vi "Control_Rack_Controler.vi"(0 "Times":dbl[](array[numeric]), 1 "Voltages Toroidal (Keep below |10|)":dbl[](array[numeric]), 2 "Voltages Helical (Keep below |10|)":dbl[](array[numeric]), 3 "error out":errorcluster, 4 "Data out 2":T1) -> (5 "error out 2":errorcluster, 6 "Data out":T1)   [LabVIEW 2017]
uses:
  Type_Defs/Data.ctl
  Type_Defs/Diagnostics.ctl
  Type_Defs/Systems.ctl
  <vilib>/DAQmx/write.llb/DAQmx Write (Analog DBL 1Chan 1Samp).vi
  <vilib>/DAQmx/create/channels.llb/DAQmx Create Channel (AO-Voltage-Basic).vi
  <vilib>/DAQmx/miscellaneous.llb/DAQmx Fill In Error Info.vi
  <vilib>/express/express shared/transition.llb/Dynamic To Waveform Array.vi
  <vilib>/express/express signal manip/GetorSetDDTAttributes/Set DDT Attributes/SetT0.vi
  <vilib>/express/express shared/transition.llb/Waveform Array To Dynamic.vi
  <vilib>/express/express signal manip/GetorSetDDTAttributes/Set DDT Attributes/Set DDT Properties.xnode
panel:
  out "hel_cur":dynamicdata(graph) caption="Helix Current Feedback"
  out "hel_vol":dynamicdata(graph) caption="Helix Voltage Feedback"
  out "hel_cur_set":dynamicdata(graph) caption="Helix Limited Current Set Point"
  out "torr_cur_set":dynamicdata(graph) caption="Torroidal Limited Current Set Point"
  out "torr_vol":dynamicdata(graph) caption="Torroidal Voltage Feedback"
  out "torr_cur":dynamicdata(graph) caption="Torroidal Current Feedback"
  out "Voltage Toroidal":dbl
  out "Time":dbl
  out "Voltage Helical":dbl
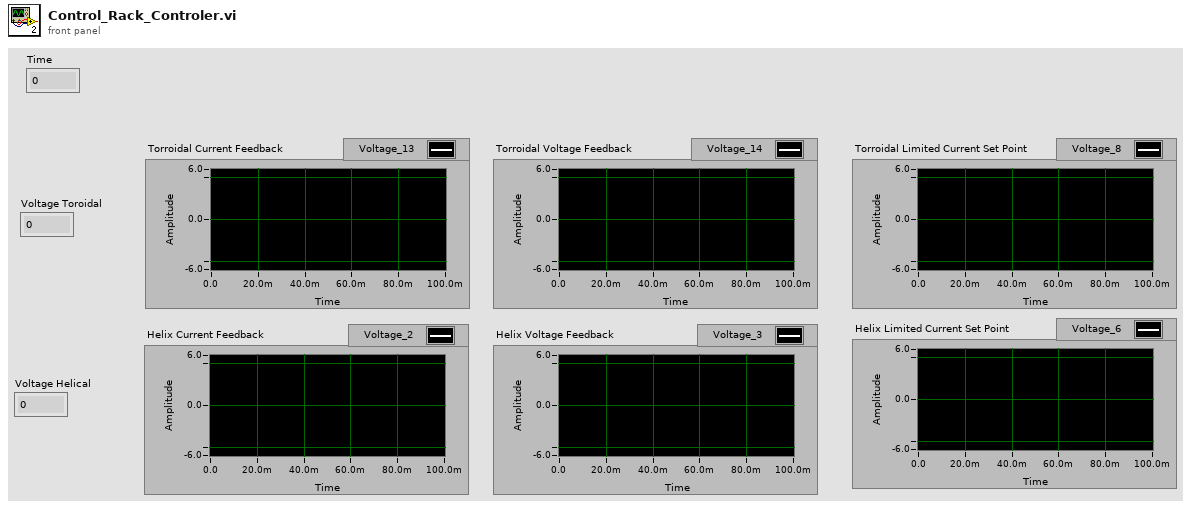
[diagram p1: front panel]
types:
  T1 = typedef "Data.ctl" = cluster{"User Name":string, "Experiment Number":i32, "Start Time":timestamp, "Data":dbl[], "Step Number":i32, "Step Instructions":string, "Diagnostics":T2, "Experiment Purpose":string, "Experiment State":enum16{"Off", "Setting Up", "Ready", "In Progress", "Shutting Down"}, "Systems":T3, "Vacuum Pressure":dbl, "Fieldpoints":cluster{"System Boolean Fieldpoints":cluster{"Compressed Air":refnum<k21>, "T-20kV Power Switch":refnum<k21>, "T-Rectifier":refnum<k21>, "Engage Interlock":refnum<k21>, "Ventilator":refnum<k21>, "Magnetron":refnum<k21>, "H-20kV Power Switch":refnum<k21>, "H-Rectifier":refnum<k21>, "Main Water Pump":refnum<k21>, "WEGA Water Pump":refnum<k21>, "Gas Inlet Valves":refnum<k21>}, "Step Fieldpoints":cluster{"Exhaust Ventillator":refnum<k21>, "Compressed Air":refnum<k21>, "Water Pressure":refnum<k21>, "Interlock":refnum<k21>, "Toroidal Power Supply 1":refnum<k21>, "Toroidal Power Supply 2":refnum<k21>, "Toroidal Rectifier":refnum<k21>, "Helical Power Supply":refnum<k21>, "Helical Rectifier":refnum<k21>, "6kW Magnetron Standby":refnum<k21>, "20kW Magnetron Standby":refnum<k21>}}, "Pressure History":cluster{"Seconds into Experiment":i32[], "Pressure Data":dbl[]}, "Time Computer Control":dbl[], "Toroidal Voltage Computer Control":dbl[], "Helical Voltage Computer Control":dbl[], "Toroidal Current":dbl[], "Toroidal Voltage":dbl[], "Toroidal Current Set Point":dbl[], "Helical Current Set Point":dbl[], "Helical Voltage":dbl[], "Helical Current":dbl[], "Experiment Folder":path, "Run Another Shot?":bool}
  T2 = typedef "Diagnostics.ctl" = cluster{"Langmuir Probe":bool, "Rogowski 1":bool, "Rogowski 2":bool, "Rogowski 3":bool, "B-dot 1":bool, "B-dot 2":bool}
  T3 = typedef "Systems.ctl" = cluster{"Compressed Air":bool, "T-20kV Power Switch":bool, "T-Rectifier":bool, "Engage Interlock":bool, "Ventilator":bool, "Magnetron":bool, "H-20kV Power Switch":bool, "H-Rectifier":bool, "Main Water Pump":bool, "WEGA Water Pump":bool, "Gas Inlet Valves":bool}
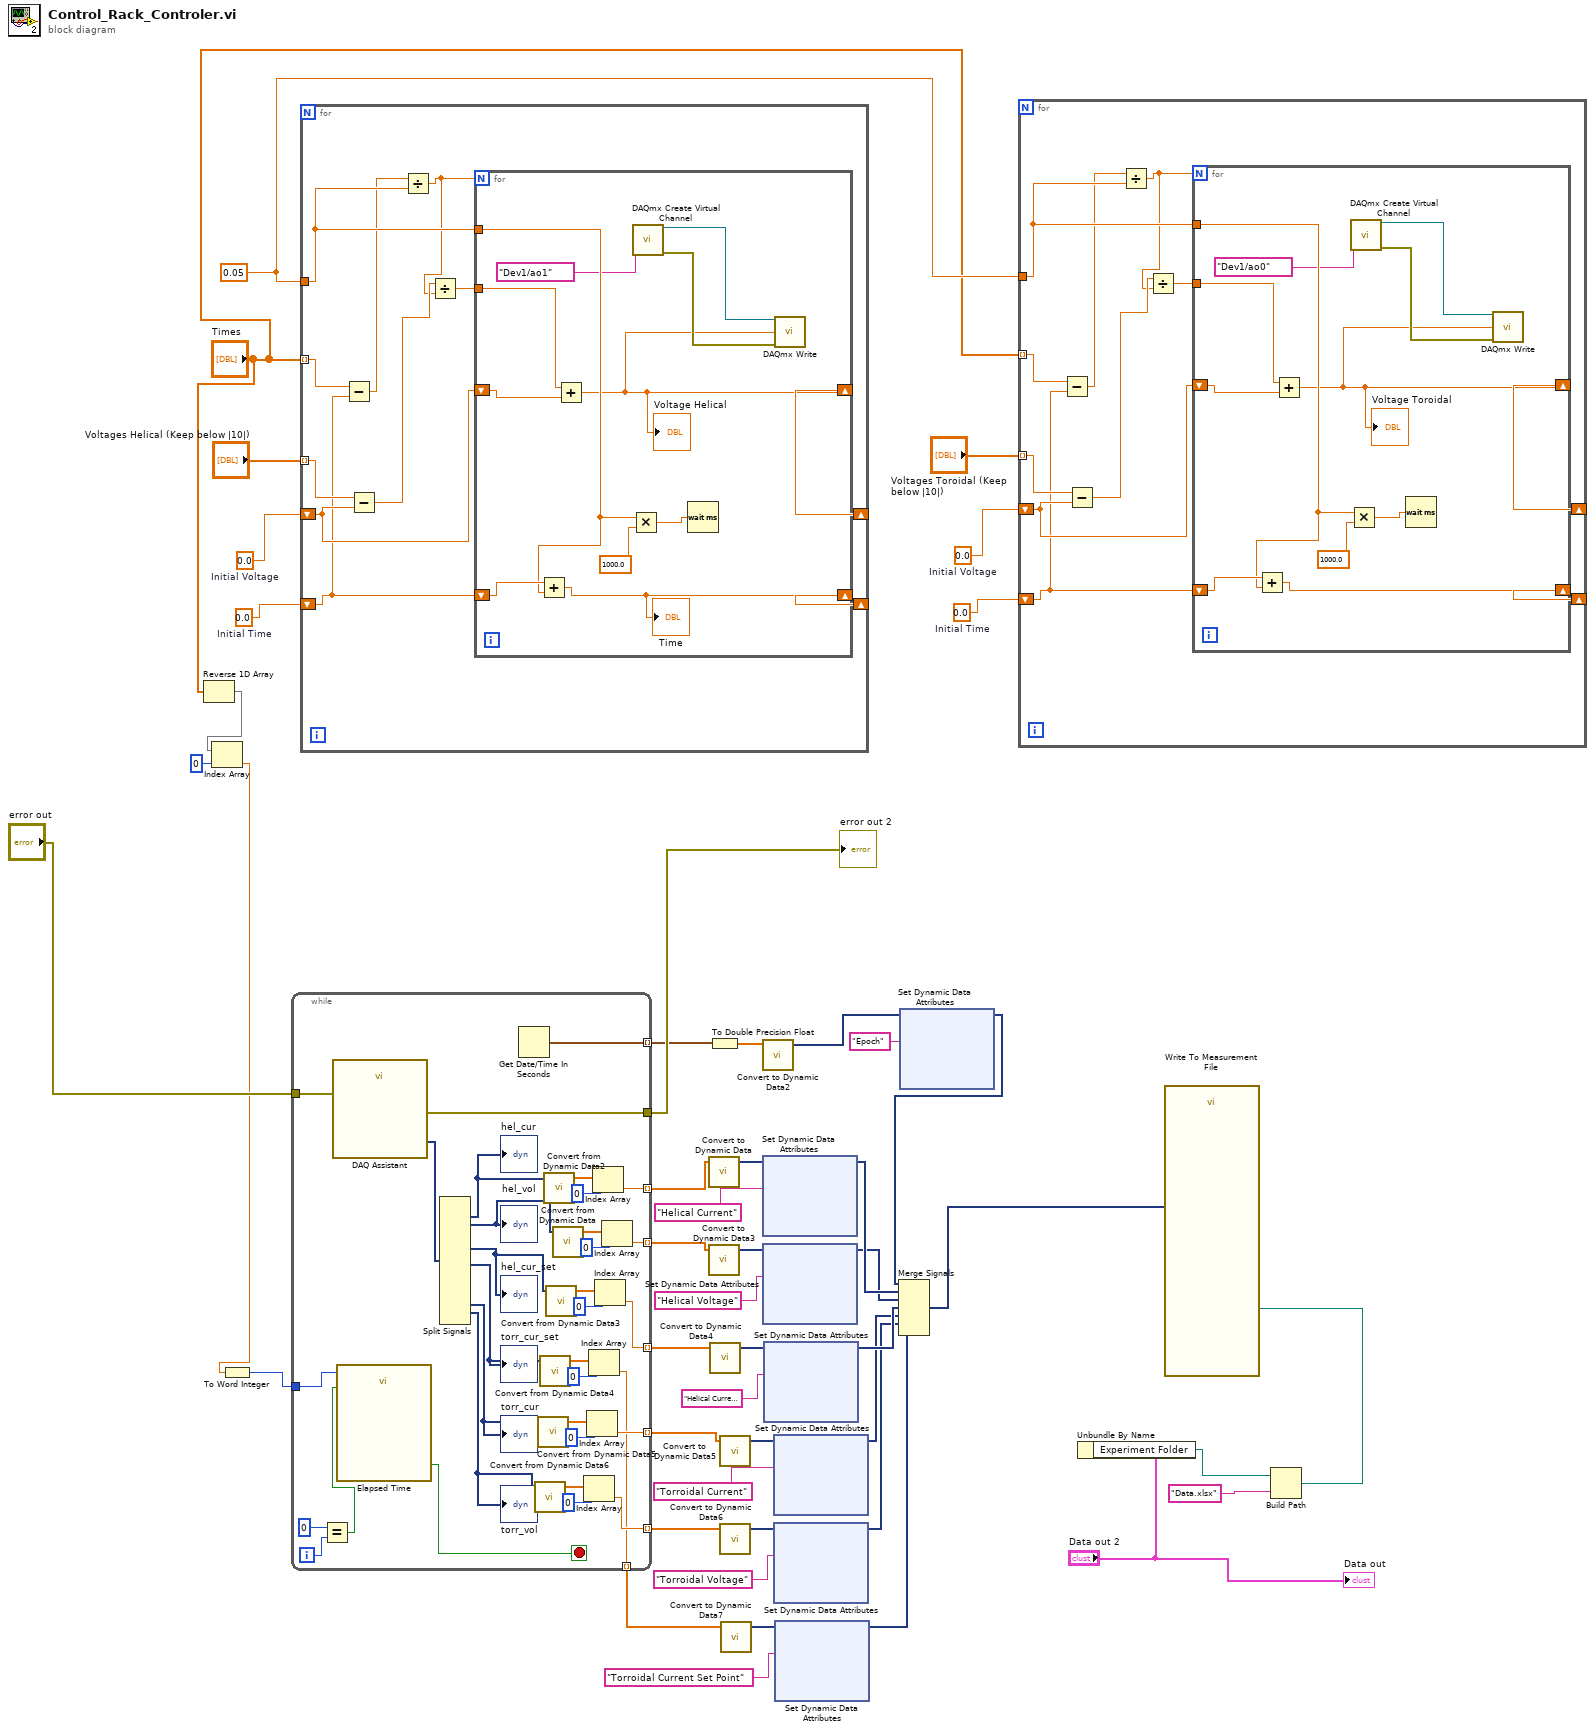
[diagram p0: block diagram]
diagram:
  w42 = 0.05 ("Timestep (in seconds, keep above 1/20s)")
  w45 = 0.0  # Initial Time
  w44 = 0.0  # Initial Voltage
  w46 = 0.0  # Initial Time
  w47 = 0.0  # Initial Voltage
  n1 = Reverse 1D Array(array="Times") -> (reversed array=w40:dbl[])
  n2 = Index Array(array=w40, index=0) -> (element=w36:dbl)
  n3 = To Word Integer(number=w36) -> (16bit integer=w35:i16)
  n4 = while {
    tunnel: "error out" -> [w80]
    tunnel: [w79] -> w37
    tunnel: w35 -> [w77]
    tunnel: [w73] -> w29 mode=indexing
    tunnel: [w72] -> w27 mode=indexing
    tunnel: [w56] -> w5 mode=indexing
    tunnel: [w55] -> w4 mode=indexing
    tunnel: [w54] -> w3 mode=indexing
    tunnel: [w53] -> w2 mode=indexing
    tunnel: [w52] -> w1 mode=indexing
    i -> [w51]
    stop <- w78 stop-if-true
    n5 = Equal?(x=0, y=w51) -> (x = y?=w49:bool)
    n6 = call "DAQ Assistant"("error in"=w80) -> ("data"=w81:dynamicdata, "error out"=w79:errorcluster)  [unwired: 16 in, 1 out]
    n7 = call "Elapsed Time"("Time Target (s)"=w77, "Reset"=w49) -> ("Time has Elapsed"=w78:bool)  [unwired: 10 in, 7 out]
    n8 = Split Signals(w81) -> (w76:dynamicdata, w61:dynamicdata, w60:dynamicdata, w59:dynamicdata, w58:dynamicdata, w57:dynamicdata)  [unwired: 16 in, 10 out]
    "hel_cur" <- w76
    "hel_vol" <- w61
    "hel_cur_set" <- w60
    "torr_cur_set" <- w59
    "torr_vol" <- w57
    "torr_cur" <- w58
    n9 = Get Date/Time In Seconds() -> (seconds since 1Jan1904=w72:timestamp)
    n10 = call "Convert from Dynamic Data6"("Dynamic Data Type"=w57) -> ("Array"=w63:dbl[])  [unwired: 3 in]
    n11 = call "Convert from Dynamic Data5"("Dynamic Data Type"=w58) -> ("Array"=w65:dbl[])  [unwired: 3 in]
    n12 = call "Convert from Dynamic Data4"("Dynamic Data Type"=w59) -> ("Array"=w67:dbl[])  [unwired: 3 in]
    n13 = call "Convert from Dynamic Data2"("Dynamic Data Type"=w76) -> ("Array"=w75:dbl[])  [unwired: 3 in]
    n14 = call "Convert from Dynamic Data3"("Dynamic Data Type"=w60) -> ("Array"=w69:dbl[])  [unwired: 3 in]
    n15 = call "Convert from Dynamic Data"("Dynamic Data Type"=w61) -> ("Array"=w71:dbl[])  [unwired: 3 in]
    n16 = Index Array(array=w63, index=0) -> (element=w53:dbl)
    n17 = Index Array(array=w65, index=0) -> (element=w54:dbl)
    n18 = Index Array(array=w67, index=0) -> (element=w52:dbl)
    n19 = Index Array(array=w75, index=0) -> (element=w73:dbl)
    n20 = Index Array(array=w69, index=0) -> (element=w55:dbl)
    n21 = Index Array(array=w71, index=0) -> (element=w56:dbl)
  }
  "error out 2" <- w37
  n22 = for {
    tunnel: "Voltages Helical (Keep below |10|)" -> [w92] mode=indexing
    tunnel: "Times" -> [w85] mode=indexing
    tunnel: w42 -> [w87]
    shift-right: [w88] -> _
    shift-left: w47 -> [w91]
    shift-right: [w86] -> _
    shift-left: w46 -> [w84]
    n23 = Subtract(x=w85, y=w84) -> (x-y=w83:dbl)
    n24 = Subtract(x=w92, y=w91) -> (x-y=w90:dbl)
    n25 = Divide(x=w83, y=w87) -> (x/y=w82:dbl)
    n26 = Divide(x=w90, y=w82) -> (x/y=w89:dbl)
    n27 = for {
      N: w82 -> [_]
      shift-right: [w93] -> w88
      shift-left: w91 -> [w103]
      tunnel: w89 -> [w102]
      tunnel: w87 -> [w99]
      shift-right: [w97] -> w86
      shift-left: w84 -> [w101]
      n28 = Add(x=w101, y=w99) -> (x+y=w97:dbl)
      "Time" <- w97
      n29 = Add(x=w102, y=w103) -> (x+y=w93:dbl)
      "Voltage Helical" <- w93
      n30 = Multiply(x=w99, y=1000.0) -> (x*y=w100:dbl)
      n31 = call-poly <vilib>:"DAQmx Create Virtual Channel.vi"("physical channels"=tag "Dev1/ao1" ("write channel (torr = ao0, hel = ao1)")) -> ("task out"=w94:refnum<k21>, "error out"=w95:errorcluster)  [unwired: 13 in]
      n32 = Wait (ms)(milliseconds to wait=w100) -> ()  [unwired: 1 out]
      n33 = call-poly <vilib>:"DAQmx Write.vi"("task/channels in"=w94, "data"=w93, "error in"=w95) -> ()  [unwired: 10 in, 3 out]
    }
  }
  n34 = call "Convert to Dynamic Data"("Array"=w29) -> ("Dynamic Data Type"=w30:dynamicdata)  [unwired: 3 in]
  n35 = call "Convert to Dynamic Data3"("Array"=w5) -> ("Dynamic Data Type"=w20:dynamicdata)  [unwired: 3 in]
  n36 = To Double Precision Float(number=w27) -> (double precision float=w26:dbl[])
  n37 = call "Convert to Dynamic Data4"("Array"=w4) -> ("Dynamic Data Type"=w19:dynamicdata)  [unwired: 3 in]
  n38 = call "Convert to Dynamic Data5"("Array"=w3) -> ("Dynamic Data Type"=w18:dynamicdata)  [unwired: 3 in]
  n39 = call "Convert to Dynamic Data6"("Array"=w2) -> ("Dynamic Data Type"=w16:dynamicdata)  [unwired: 3 in]
  n40 = call "Convert to Dynamic Data7"("Array"=w1) -> ("Dynamic Data Type"=w15:dynamicdata)  [unwired: 3 in]
  n41 = call "Convert to Dynamic Data2"("Array"=w26) -> ("Dynamic Data Type"=w25:dynamicdata)  [unwired: 3 in]
  n42 = xnode "Set Dynamic Data Attributes"("Signals In"=w30, "Signal Name"="Helical Current") -> ("Signals Out"=w23:dynamicdata)  [unwired: 2 in, 1 out]
  n43 = xnode "Set Dynamic Data Attributes"("Signals In"=w20, "Signal Name"="Helical Voltage") -> ("Signals Out"=w14:dynamicdata)  [unwired: 2 in, 1 out]
  n44 = xnode "Set Dynamic Data Attributes"("Signals In"=w19, "Signal Name"="Helical Current Set Point") -> ("Signals Out"=w13:dynamicdata)  [unwired: 2 in, 1 out]
  n45 = xnode "Set Dynamic Data Attributes"("Signals In"=w18, "Signal Name"="Torroidal Current") -> ("Signals Out"=w12:dynamicdata)  [unwired: 2 in, 1 out]
  n46 = xnode "Set Dynamic Data Attributes"("Signals In"=w16, "Signal Name"="Torroidal Voltage") -> ("Signals Out"=w11:dynamicdata)  [unwired: 2 in, 1 out]
  n47 = xnode "Set Dynamic Data Attributes"("Signals In"=w15, "Signal Name"="Torroidal Current Set Point") -> ("Signals Out"=w10:dynamicdata)  [unwired: 2 in, 1 out]
  n48 = xnode "Set Dynamic Data Attributes"("Signals In"=w25, "Signal Name"="Epoch") -> ("Signals Out"=w22:dynamicdata)  [unwired: 2 in, 1 out]
  n49 = Merge Signals(w22, w23, w14, w13, w12, w11, w10) -> (w21:dynamicdata)
  n50 = for {
    tunnel: "Voltages Toroidal (Keep below |10|)" -> [w114] mode=indexing
    tunnel: "Times" -> [w107] mode=indexing
    tunnel: w42 -> [w109]
    shift-right: [w110] -> _
    shift-left: w44 -> [w113]
    shift-right: [w108] -> _
    shift-left: w45 -> [w106]
    n51 = Subtract(x=w107, y=w106) -> (x-y=w105:dbl)
    n52 = Subtract(x=w114, y=w113) -> (x-y=w112:dbl)
    n53 = Divide(x=w105, y=w109) -> (x/y=w104:dbl)
    n54 = Divide(x=w112, y=w104) -> (x/y=w111:dbl)
    n55 = for {
      N: w104 -> [_]
      shift-right: [w115] -> w110
      shift-left: w113 -> [w125]
      tunnel: w111 -> [w124]
      tunnel: w109 -> [w121]
      shift-right: [w119] -> w108
      shift-left: w106 -> [w123]
      n56 = Add(x=w123, y=w121) -> (x+y=w119:dbl)
      n57 = Add(x=w124, y=w125) -> (x+y=w115:dbl)
      "Voltage Toroidal" <- w115
      n58 = Multiply(x=w121, y=1000.0) -> (x*y=w122:dbl)
      n59 = call-poly <vilib>:"DAQmx Create Virtual Channel.vi"("physical channels"=tag "Dev1/ao0" ("write channel (torr = ao0, hel = ao1) 2")) -> ("task out"=w116:refnum<k21>, "error out"=w117:errorcluster)  [unwired: 13 in]
      n60 = Wait (ms)(milliseconds to wait=w122) -> ()  [unwired: 1 out]
      n61 = call-poly <vilib>:"DAQmx Write.vi"("task/channels in"=w116, "data"=w115, "error in"=w117) -> ()  [unwired: 10 in, 3 out]
    }
  }
  n62 = Unbundle By Name("Data out 2") -> ("Experiment Folder"=w32:path)
  n63 = Build Path(base path=w32, name or relative path="Data.xlsx") -> (appended path=w33:path)
  n64 = call "Write To Measurement File"("Signals"=w21, "Filename"=w33) -> ()  [unwired: 15 in, 3 out]
  "Data out" <- "Data out 2"
